vi "Cannon Get and use.vi"(1 "Move":dbl, 2 "InTake Max":bool, 3 "Fire":bool) -> (0 "Cannon Info":T1)   [LabVIEW 2013]
uses:
  Kick Global.vi
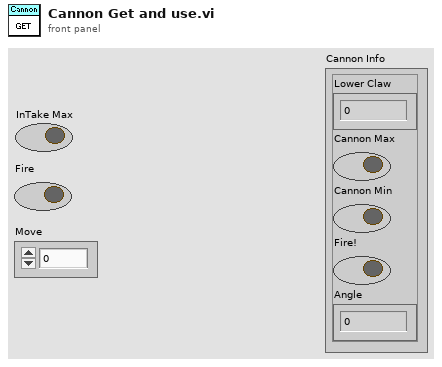
[diagram p1: front panel]
types:
  T1 = cluster{"Lower Claw":dbl, "Cannon Max":bool, "Cannon Min":bool, "Fire!":bool, "Angle":dbl}
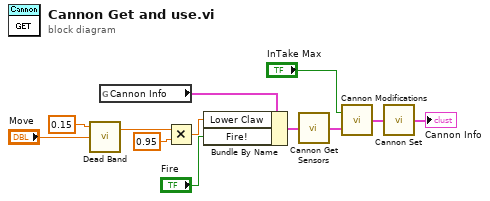
[diagram p0: block diagram]
diagram:
  n1 = call "Dead Band.vi"("Axis 1 In"="Move", "Dead Band"=0.15) -> ("Axis 1 Out"=w4:dbl)  [unwired: 1 in, 1 out]
  n2 = global read "Kick Global.vi" "Cannon Info"() -> (w12:T1)
  n3 = Multiply(x=w4, y=0.95) -> (x*y=w2:dbl)
  n4 = Bundle By Name(cluster=w12, "Lower Claw"=w2, "Fire!"="Fire") -> (w8:T1)
  n5 = call "Cannon Get Sensors.vi"("Cannon Info"=w8) -> ("Cannon Info"=w10:T1)
  n6 = call "Cannon Modifications.vi"("Cannon Info"=w10, "InTake Max"="InTake Max") -> ("Cannon Info"=w9:T1)
  n7 = call "Cannon Set.vi"("Cannon Info"=w9) -> ("Cannon Info"=→"Cannon Info":T1)
